vi "GetType.vi"(8 "error in (no error)":errorcluster, 11 "Write Beep Parameters Msg":refnum<class "Write Beep Parameters Msg.lvclass">) -> (0 "error out":errorcluster, 2 "Data Sample":variant, 3 "Write Beep Parameters Msg":refnum<class "Write Beep Parameters Msg.lvclass">)   [LabVIEW 2016, in "CS++BeepActor.lvlib" / "Write Beep Parameters Msg.lvclass"]
uses:
  Write Beep Parameters Msg.lvclass
  Write Beep Parameters Msg.lvclass/Write Beep Parameters Msg.ctl
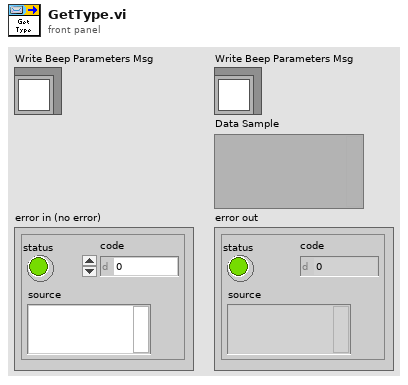
[diagram p1: front panel]
types:
  T1 = cluster{"Frequency (440)":dbl[unit], "Duration":dbl[unit], "Use System Alert?":bool}
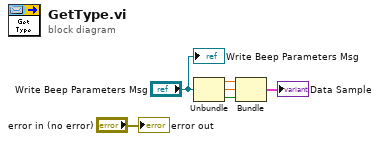
[diagram p0: block diagram]
diagram:
  n1 = Unbundle("Write Beep Parameters Msg") -> (w3:dbl[unit], w2:dbl[unit], w1:bool)
  n2 = Bundle("Frequency (440)"=w3, "Duration"=w2, "Use System Alert?"=w1) -> (→"Data Sample":T1)  [unwired: 1 in]
  "error out" <- "error in (no error)"
  "Write Beep Parameters Msg" <- "Write Beep Parameters Msg"
